vi "Memory.Array.Set Pointer.vi"(8 "error in (no error)":errorcluster, 10 "Pointer":refnum<class "Memory.Pointer.Void.lvclass">, 11 "Array in":refnum<class "Memory.Array.Void.lvclass">) -> (0 "error out":errorcluster, 3 "Array out":refnum<class "Memory.Array.Void.lvclass">)   [LabVIEW 2016, in "LabVIEW Memory Manager.lvlib" / "Memory.Array.Void.lvclass"]
uses:
  Memory.Array.Void.lvclass
  Pointer/Pointer.Void/Memory.Pointer.Void.lvclass
  Memory.Array.Void.lvclass/Memory.Array.Void.ctl
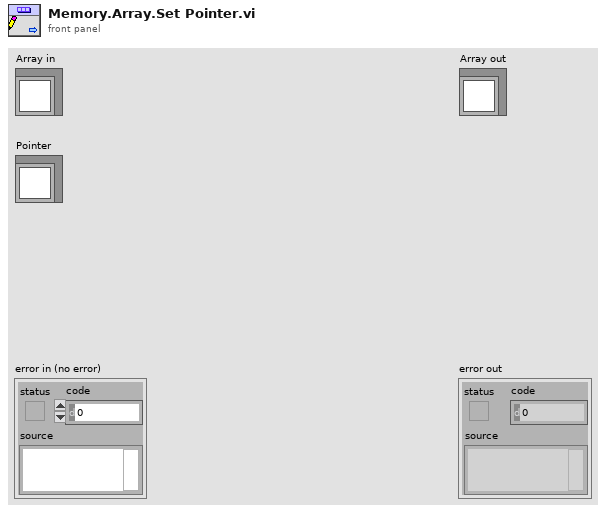
[diagram p1: front panel]
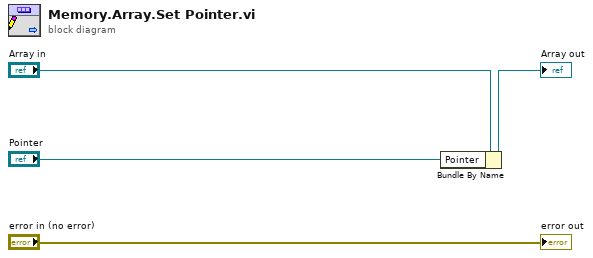
[diagram p0: block diagram]
diagram:
  n1 = Bundle By Name(cluster="Array in", "Pointer"="Pointer") -> (→"Array out":refnum<class "Memory.Array.Void.lvclass">)
  "error out" <- "error in (no error)"
